vi "test_count3.vi"() -> ()   [LabVIEW 2013]
uses:
  <instrlib>/_niInstr/Basic Elements/v1/FPGA/Private/Count Down U32.vi
  <instrlib>/_niInstr/Basic Elements/v1/FPGA/niInstr Basic Elements v1 FPGA.lvlib
panel:
  out "Waveform Graph 4":i16[][](graph)
  out "Waveform Graph 3":i16[][](graph)
  out "Waveform Graph 2":u32[](graph)
  out "counting":bool
  out "output valid":bool
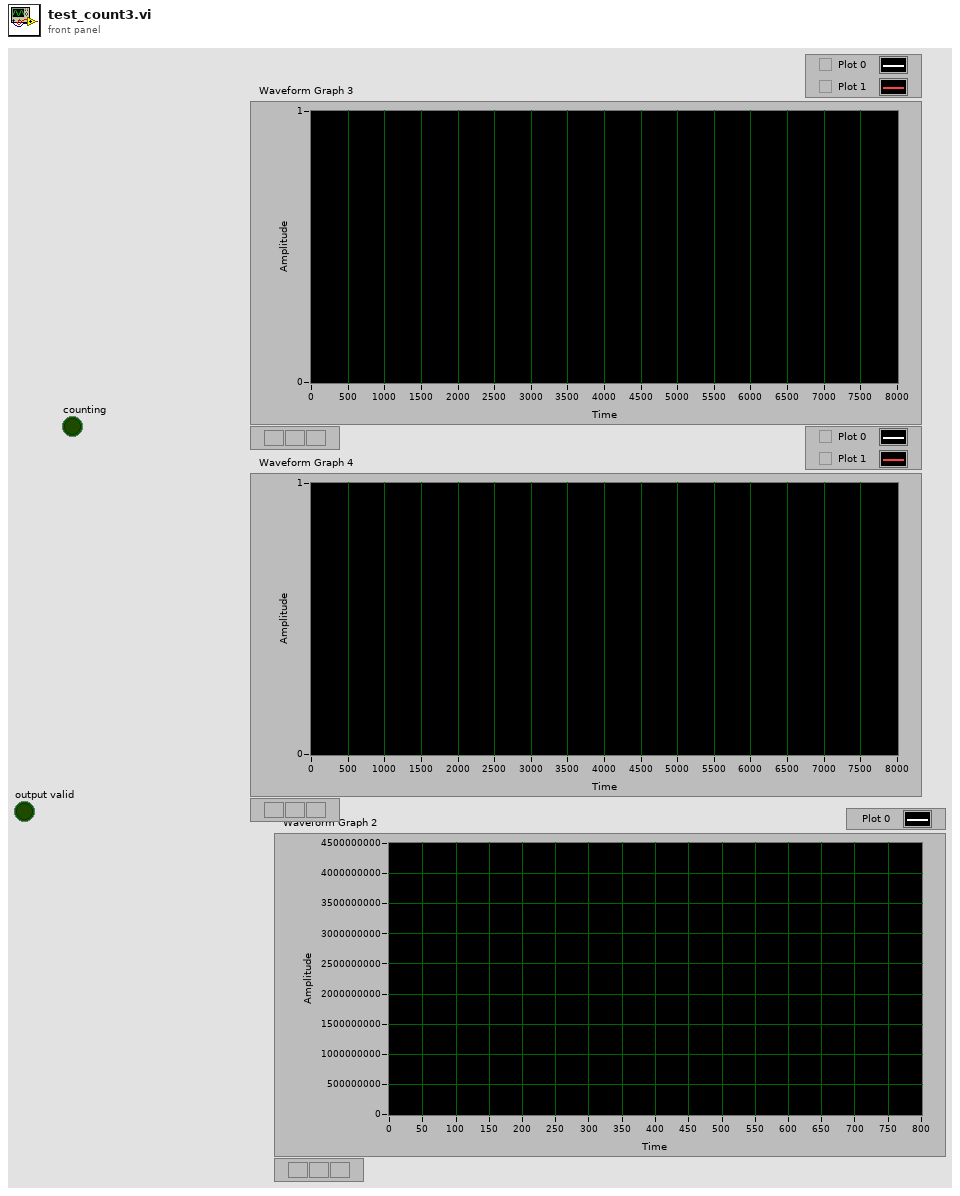
[diagram p1: front panel]
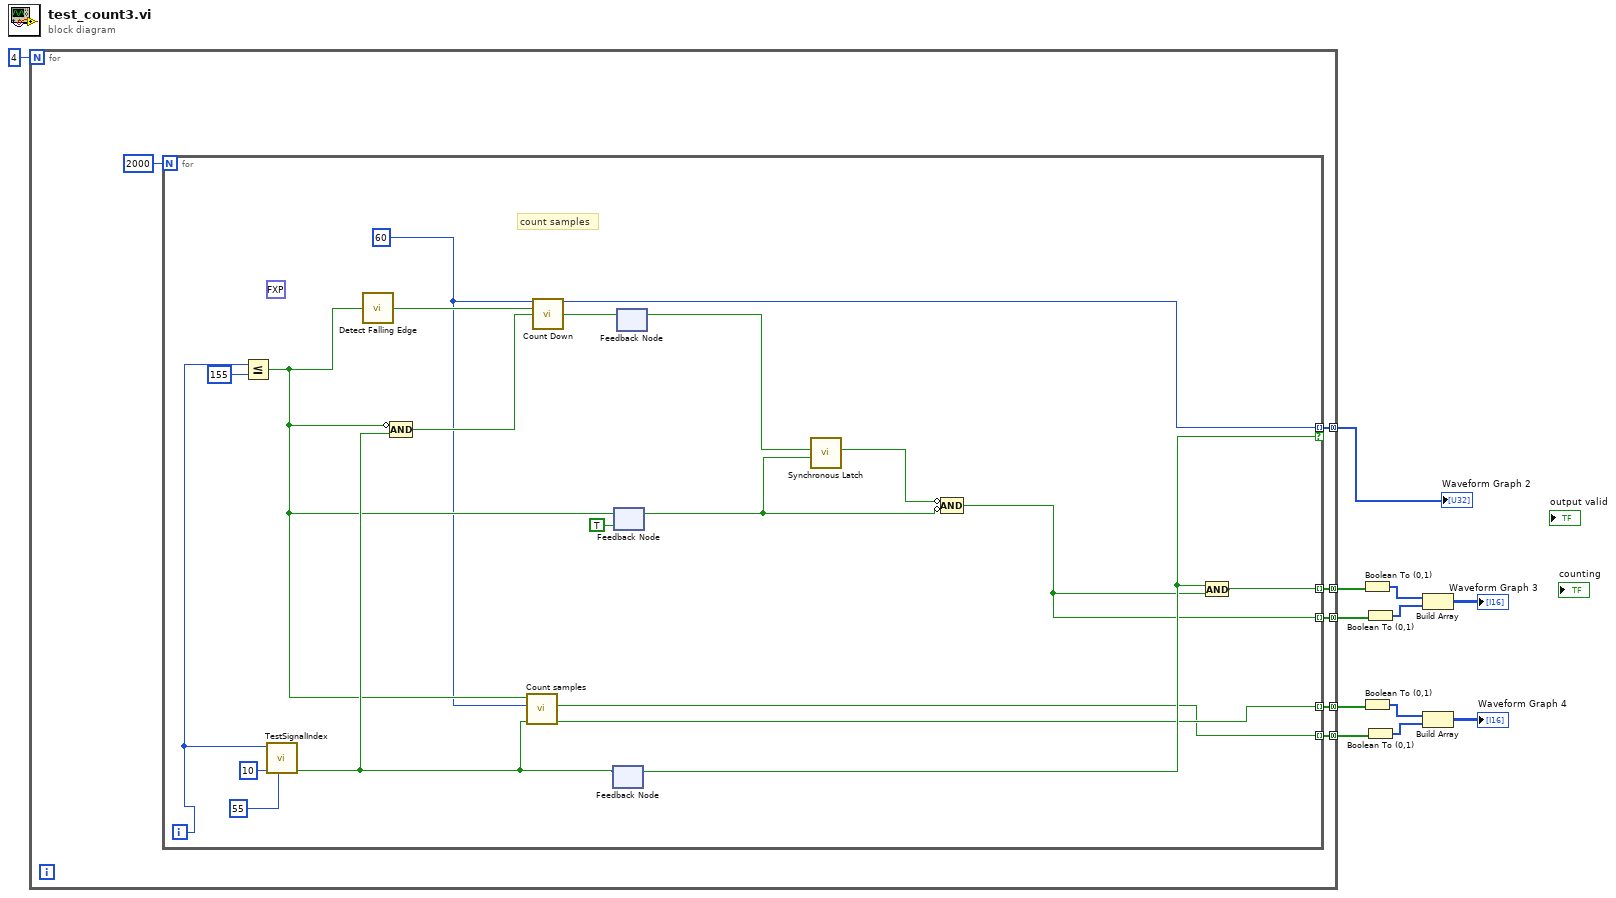
[diagram p0: block diagram]
diagram:
  n1 = for {
    N: 4 -> [_]
    tunnel: [w17] -> w12 mode=concatenating
    tunnel: [w16] -> w11 mode=concatenating
    tunnel: [w15] -> w9 mode=concatenating
    tunnel: [w13] -> w1 mode=concatenating
    tunnel: [w14] -> w2 mode=concatenating
    n2 = for {
      N: 2000 -> [_]
      tunnel: [w29] -> w17 mode=indexing
      tunnel: [w33] -> w16 mode=indexing if=w32
      tunnel: [w21] -> w15 mode=indexing
      tunnel: [w27] -> w13 mode=indexing
      tunnel: [w26] -> w14 mode=indexing
      i -> [w36]
      w19 = u32 60 ("count in")
      (unwired) fxp<+/-,16,16> 60.0 ("t")
      # "count samples"
      n3 = Less Or Equal?(x=w36, y=155) -> (x <= y?=w25:bool)
      n4 = call "TestSignalIndex.vi"("initial delay"=55, "cycles per sample"=10, "index"=w36) -> ("valid out"=w30:bool)  [unwired: 7 in, 1 out]
      n5 = call <instrlib>:"Detect Falling Edge.vi"("signal"=w25) -> ("edge detected"=w34:bool)  [unwired: 14 in]
      n6 = Compound Arithmetic op=AND(invert w25, w30) -> (w28:bool)
      n7 = call "Count samples.vi"("input valid"=w30, "number to count"=w19, "Reset"=w25) -> ("output valid"=w27:bool, "counting"=w26:bool)  [unwired: 7 in]
      n8 = call-poly <instrlib>:"Count Down.vi"("count in"=w19, "load"=w34, "decrement"=w28) -> ("count out"=w33:u32, "terminal count"=w24:bool)  [unwired: 11 in]
      n9 = feedback #1() -> (w32:bool)  [unwired: 1 in]
      n10 = feedback-in #1(w30) -> ()
      n11 = feedback #2(TRUE) -> (w22:bool)
      n12 = feedback-in #2(w25) -> ()
      n13 = feedback-in #3(w24) -> ()
      n14 = feedback #3() -> (w23:bool)  [unwired: 1 in]
      n15 = call <instrlib>:"Synchronous Latch.vi"("clear"=w22, "set"=w23) -> ("out"=w20:bool)  [unwired: 9 in]
      n16 = Compound Arithmetic op=AND(invert w20, invert w22) -> (w21:bool)
      n17 = And(x=w32, y=w21) -> (x .and. y?=w29:bool)
    }
  }
  "Waveform Graph 2" <- w11
  n18 = Boolean To (0,1)(Boolean=w12) -> (0, 1=w8:i16[])
  n19 = Boolean To (0,1)(Boolean=w1) -> (0, 1=w3:i16[])
  n20 = Boolean To (0,1)(Boolean=w9) -> (0, 1=w7:i16[])
  n21 = Boolean To (0,1)(Boolean=w2) -> (0, 1=w4:i16[])
  n22 = Build Array(w8, w7) -> (→"Waveform Graph 3":i16[][])
  n23 = Build Array(w3, w4) -> (→"Waveform Graph 4":i16[][])
